vi "服务器.vi"() -> ()   [LabVIEW 2017]
uses:
  <vilib>/Analysis/NI_AALBase.lvlib
panel:
  out "名称":string
  out "周期":i32
  out "波形图":dbl[](graph)
  in  "停止":bool
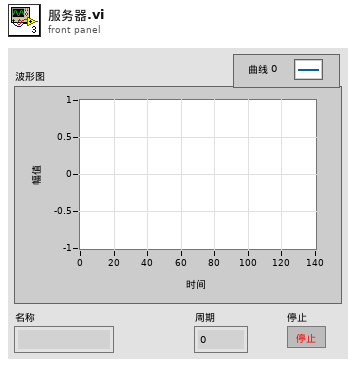
[diagram p1: front panel]
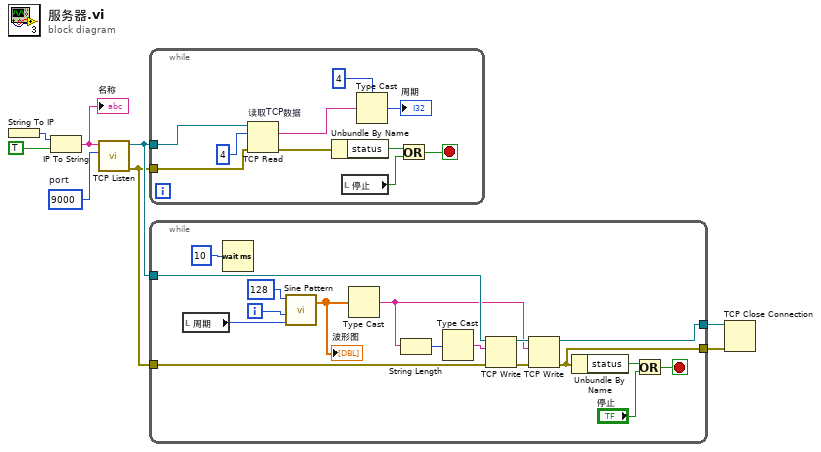
[diagram p0: block diagram]
diagram:
  w8 = u16 9000  # port
  n1 = String To IP() -> (0:w6:u32)  [unwired: 1 in]
  n2 = IP To String(1:TRUE ("句点符号？(F)"), 2:w6) -> (0:w1:string)
  "名称" <- w1
  n3 = call <vilib>:"TCP Listen.vi"("port"=w8, "service name"=w1) -> ("error out"=w2:errorcluster, "connection ID"=w3:refnum<k5>)  [unwired: 5 in, 3 out]
  n4 = while {
    tunnel: w3 -> [w18]
    tunnel: w2 -> [w15]
    stop <- w16 stop-if-true
    n5 = TCP Read "读取TCP数据"(connection ID=w18, bytes to read=4 ("读取的字节"), error in (no error)=w15) -> (data out=w10:string, error out=w11:errorcluster)  [unwired: 2 in, 1 out]
    n6 = Unbundle By Name(w11) -> ("status"=w14:bool)
    n7 = local read "停止"() -> (w17:bool)
    n8 = Type Cast(type=4, x=w10) -> (*(type *) &x=→"周期":i32)
    n9 = Or(x=w14, y=w17) -> (x .or. y?=w16:bool)
  }
  n10 = while {
    tunnel: w3 -> [w33]
    tunnel: w2 -> [w32]
    tunnel: [w35] -> w5
    tunnel: [w23] -> w4
    i -> [w26]
    stop <- w21 stop-if-true
    n11 = local read "周期"() -> (w19:i32)
    n12 = Wait (ms)(milliseconds to wait=u32 10 ("等待时间（毫秒）")) -> ()  [unwired: 1 out]
    n13 = call <vilib>:"Sine Pattern.vi"("cycles"=w19, "phase(degrees)"=w26, "samples"=128) -> ("Sinusoidal Pattern"=w25:dbl[])  [unwired: 1 in, 1 out]
    "波形图" <- w25
    n14 = Type Cast(x=w25) -> (*(type *) &x=w20:string)  [unwired: 1 in]
    n15 = String Length(string=w20) -> (length=w28:i32)
    n16 = Type Cast(x=w28) -> (*(type *) &x=w27:string)  [unwired: 1 in]
    n17 = TCP Write(connection ID=w33, data in=w27, error in (no error)=w32) -> (connection ID out=w31:refnum<k5>, error out=w30:errorcluster)  [unwired: 1 in, 1 out]
    n18 = TCP Write(connection ID=w31, data in=w20, error in (no error)=w30) -> (connection ID out=w35:refnum<k5>, error out=w23:errorcluster)  [unwired: 1 in, 1 out]
    n19 = Unbundle By Name(w23) -> ("status"=w22:bool)
    n20 = Or(x=w22, y="停止") -> (x .or. y?=w21:bool)
  }
  n21 = TCP Close Connection(connection ID=w5, error in (no error)=w4) -> ()  [unwired: 1 in, 2 out]
